vi "solar_voy Register (Packets).vi"(6 "Suppress Errors? (T)":bool=TRUE, 8 "error in (no error)":errorcluster, 9 "Override If Exists? (F)":bool, 10 "PACKETS (No HDR)":T1[](array[typedef]) {"last_time" format="%<%H:%M:%S%3u %m/%d/%y>T"}, 11 "Voyager Refnum in":T6) -> (0 "error out":errorcluster, 3 "Voyager Refnum out":T6)   [LabVIEW 2018]
doc: "This registers multiple Voyager packets. If <b>Override If Exists?</b> is true, this overrides the existing packet. If the packet ID is 0, this generates a new ID. By default the header items are automatically added to the packet."
uses:
  solar_voy_ctl Voyager Refnum.ctl
  solar_voy_def/solar_voy_def_ctl ITEM TYPE.ctl
  type/solar_type Item Type.ctl
  solar_voy_def/solar_voy_def_ctl ITEM.ctl
  solar_voy_def/solar_voy_def_ctl PACKET.ctl
  solar_voy_def/solar_voy_def_ctl PACKET_ID.ctl
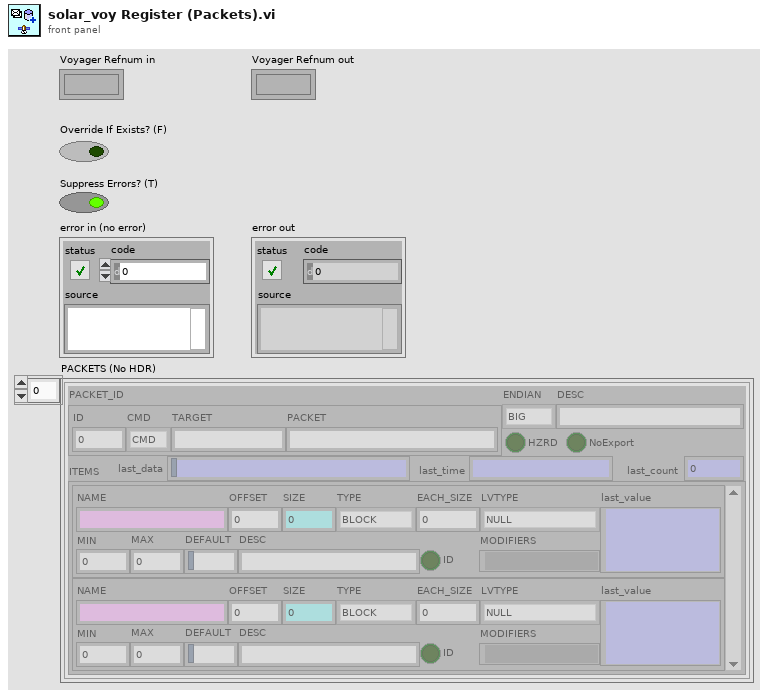
[diagram p1: front panel]
types:
  T1 = typedef "solar_voy_def_ctl PACKET.ctl" = cluster{"PACKET_ID":T2, "ENDIAN":enum8{"BIG", "LITTLE"}, "DESC":string, "HZRD":bool, "ITEMS":T3[], "NoExport":bool, "last_time":timestamp, "last_count":u32, "last_data":string}
  T2 = typedef "solar_voy_def_ctl PACKET_ID.ctl" = cluster{"ID":u16, "CMD":enum8{"CMD", "TLM"}, "TARGET":string, "PACKET":string}
  T3 = typedef "solar_voy_def_ctl ITEM.ctl" = cluster{"NAME":string, "OFFSET":i32, "SIZE":i32, "TYPE":T4, "EACH_SIZE":i32, "LVTYPE":T5, "MIN":dbl, "MAX":dbl, "DEFAULT":string, "DESC":string, "ID":bool, "MODIFIERS":variant, "last_value":variant}
  T4 = typedef "solar_voy_def_ctl ITEM TYPE.ctl" = enum8{"BLOCK", "INT", "UINT", "FLOAT", "STRING"}
  T5 = typedef "solar_type Item Type.ctl" = enum16{"NULL", "UNKNOWN", "CLUSTER", "I8", "I16", "I32", "I64", "U8", "U16", "U32", "U64", "U8_ENUM", "U16_ENUM", "U32_ENUM", "SGL", "DBL", "BOOLEAN", "STRING", "PATH", "VISA", "TAG", "TIME", "I8_1D", "I16_1D", "I32_1D", "I64_1D", "U8_1D", "U16_1D", "U32_1D", "U64_1D", "U8_ENUM_1D", "U16_ENUM_1D", "U32_ENUM_1D", "SGL_1D", "DBL_1D", "BOOLEAN_1D", "STRING_1D", "PATH_1D", "VISA_1D", "TAG_1D", "TIME_1D", "I8_2D", "I16_2D", "I32_2D", "I64_2D", "U8_2D", "U16_2D", "U32_2D", "U64_2D", "U8_ENUM_2D", "U16_ENUM_2D", "U32_ENUM_2D", "SGL_2D", "DBL_2D", "BOOLEAN_2D", "STRING_2D", "PATH_2D", "VISA_2D", "TAG_2D", "TIME_2D"}
  T6 = typedef "solar_voy_ctl Voyager Refnum.ctl" = refnum<k1>
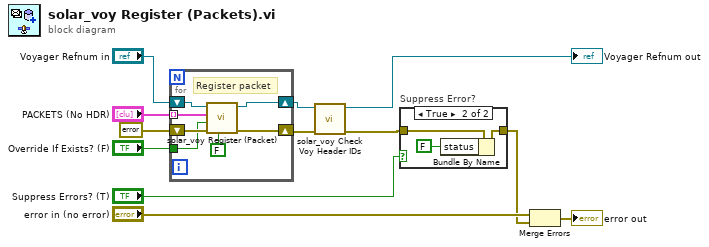
[diagram p0: block diagram]
diagram:
  n1 = for {
    tunnel: "PACKETS (No HDR)" -> [w16] mode=indexing
    shift-right: [w19] -> w4
    shift-left: errorcluster {"status"=FALSE, "code"=0, "source"=""} ("error in (no error)") -> [w18]
    tunnel: "Override If Exists? (F)" -> [w14]
    shift-right: [w13] -> w2
    shift-left: "Voyager Refnum in" -> [w15]
    # "Register packet"
    n2 = call "solar_voy Register (Packet).vi"("Suppress Errors? (T)"=FALSE, "error in (no error)"=w18, "Override If Exists? (F)"=w14, "PACKET (No HDR)"=w16, "Voyager Refnum in"=w15) -> ("error out"=w19:errorcluster, "Voyager Refnum out"=w13:T6)  [unwired: 5 in]
  }
  n3 = call "solar_voy Check Voy Header IDs.vi"("error in"=w4, "Voyager Refnum"=w2) -> ("Error out"=w3:errorcluster, "Voyager Refnum out"=→"Voyager Refnum out":T6)  [unwired: 8 in]
  n4 = case "Suppress Error?" shown="True" "Suppress Errors? (T)" {
    tunnel: w3 -> [w20 w23]
    tunnel: [w20 w22] -> w10
    frame False {
    }
    frame True {
      n5 = Bundle By Name(cluster=w23, "status"=FALSE) -> (w22:errorcluster)
    }
  }
  n6 = Merge Errors("error in (no error)", w10) -> (→"error out":errorcluster)
